vi "NN_Draw_Rectangle.vi"(4 "Clear":bool, 5 "font_size":sgl=20.0, 6 "Labels":string[](array[string])=["aeroplane", "bicycle", "bird", "boat", "bottle", "bus", "car", "cat", "chair", "cow", "diningtable", "dog", "horse", "motorbike", "person", "pottedplant", "sheep", "sofa", "train", "tvmonitor"], 7 "Border_Width":u32=4, 8 "error in (no error)":errorcluster, 9 "Colors":u32[](array[colorbox])=[6618880, 15679744, 16774656, 1740031, 13311, 33023, 52479, 65509, 65433, 65356, 65280, 5111552, 10092288, 15138560, 16763904, 16744192, 16724736, 16711680, 16711680, 16711680], 10 "Draw_Boxes":T1[](array[typedef]) {"BBox"."x" format="%#_4p"; "BBox"."y" format="%#_4p"; "BBox"."w" format="%#_4p"; "BBox"."h" format="%#_4p"}, 11 "Image_in":T3) -> (0 "error out":errorcluster, 1 "Exec_Time(s)":dbl=0.000148600014654221, 3 "Image_out":T3)   [LabVIEW 2020]
doc: "Draws bounding box regtangles around objects on the image based on BBox input information ."
uses:
  <vilib>/vision/Image Controls.llb/IMAQ Image.ctl
  <vilib>/Ngene/Deep Learning Toolkit/Toolkit/NN_Data/API/Data/Detection_Types/NN_BBox_Detection.ctl
  <vilib>/Ngene/Deep Learning Toolkit/Toolkit/NN_Data/API/Data/Detection_Types/NN_BBox.ctl
  <vilib>/Ngene/Deep Learning Toolkit/Toolkit/NN_Data/API/NN_Dims(C,H,W).ctl
  <vilib>/Ngene/Deep Learning Toolkit/Toolkit/Deep_Learning_Toolkit_by_Ngene.lvlib
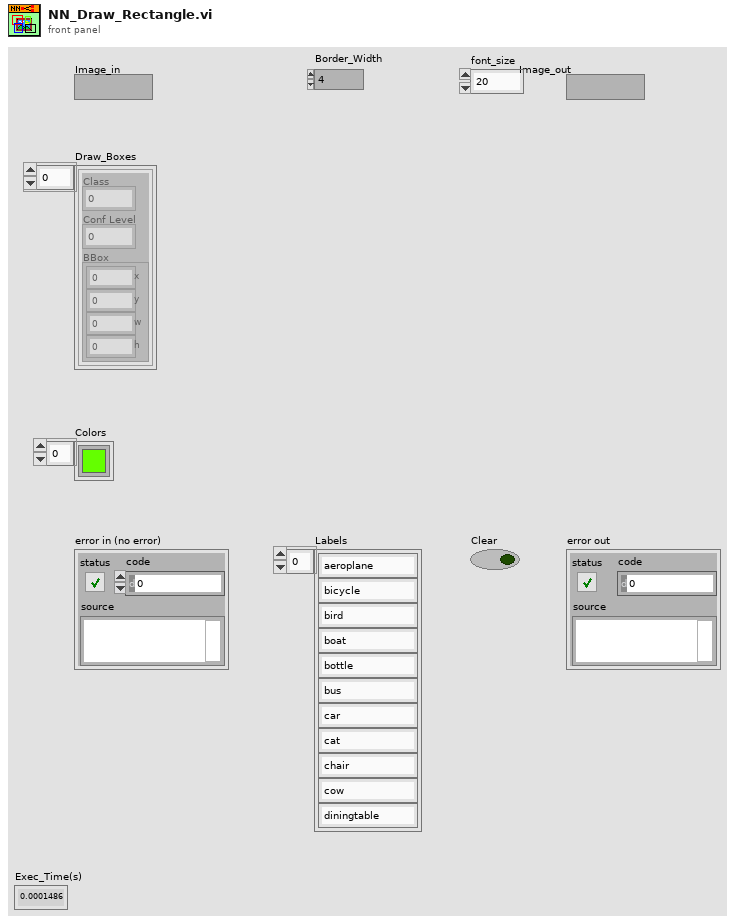
[diagram p1: front panel]
types:
  T1 = typedef "Deep_Learning_Toolkit_by_Ngene.lvlib/NN_BBox_Detection.ctl" = cluster{"Class":i32, "Conf Level":sgl, "BBox":T2}
  T2 = typedef "Deep_Learning_Toolkit_by_Ngene.lvlib/NN_BBox.ctl" = cluster{"x":sgl, "y":sgl, "w":sgl, "h":sgl}
  T3 = typedef "IMAQ Image.ctl" = refnum<image>
  T4 = typedef "Deep_Learning_Toolkit_by_Ngene.lvlib/NN_Dims(C,H,W).ctl" = cluster{"C":i32, "H":i32, "W":i32}
  T5 = cluster{"Desired Font (Application)":enum16{"User-specified Font", "Application Font", "System Font", "Dialog Font"}, "[User-specified Font]":cluster{"Font Name":string, "Size":i16, "Strikeout?":bool, "Italic?":bool, "Underline?":bool, "Outline?":bool, "Shadow?":bool, "Bold?":bool, "Rotation Angle":dbl}, "Horizontal Alignment":i16, "Vertical Alignment":i16}
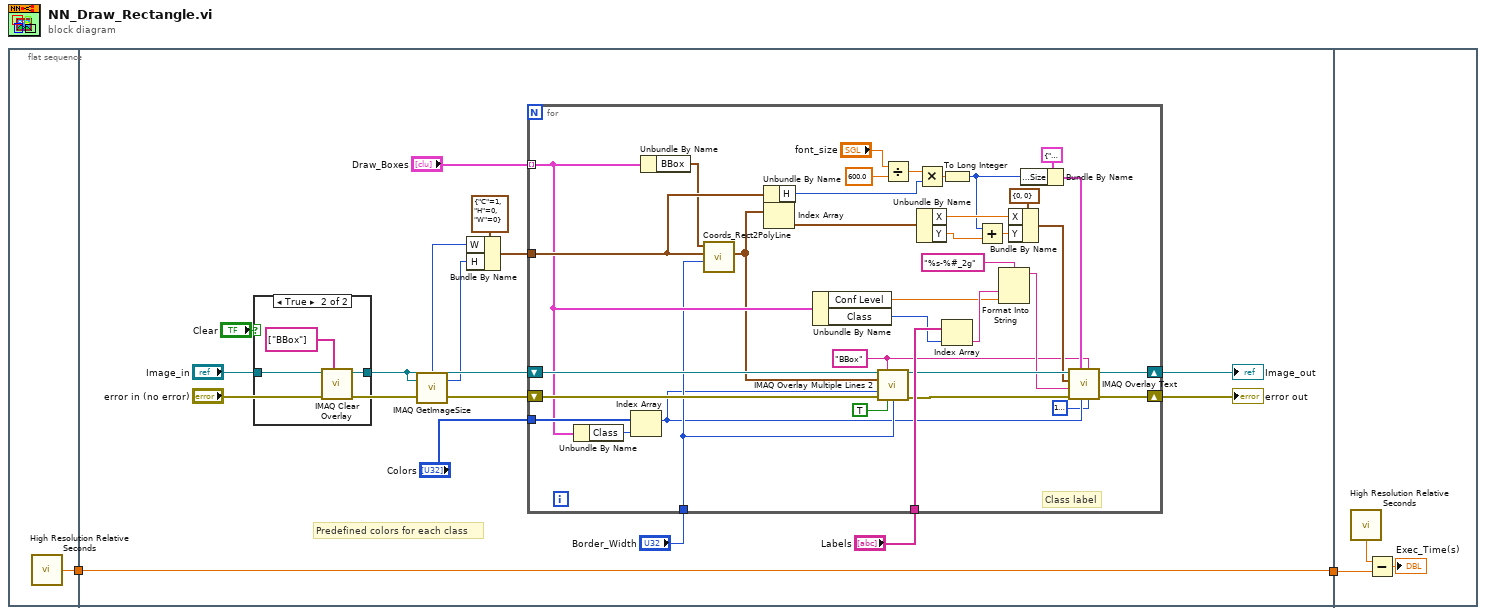
[diagram p0: block diagram]
diagram:
  n1 = flat-sequence {
    tunnel: [w3] -> w2
    tunnel: w2 -> [w9]
    tunnel: [w9] -> w1
    tunnel: w1 -> [w63]
    frame #0 {
      n2 = call <vilib>:"High Resolution Relative Seconds.vi"() -> ("relative seconds"=w3:dbl)
    }
    frame #1 {
      # "Predefined colors for each class"
      n3 = case shown="True" "Clear" {
        tunnel: "Image_in" -> [w20 w23]
        tunnel: [w20 w22] -> w12
        frame False {
        }
        frame True {
          n4 = call "IMAQ Clear Overlay"("Groups"=string[] ["BBox"], "Image"=w23) -> ("Image Out"=w22:T3)  [unwired: 8 in, 1 out]
        }
      }
      n5 = call "IMAQ GetImageSize"("Image"=w12, "error in (no error)"="error in (no error)") -> ("Y Resolution"=w10:i32, "X Resolution"=w11:i32, "error out"=w13:errorcluster)  [unwired: 2 in]
      n6 = Bundle By Name(cluster=T4 {"C"=1, "H"=0, "W"=0} ("In_Dims"), "W"=w11, "H"=w10) -> (w15:T4)
      n7 = for {
        tunnel: "Colors" -> [w60]
        shift-right: [w59] -> w19
        shift-left: w13 -> [w56]
        shift-right: [w58] -> w4
        shift-left: w12 -> [w55]
        tunnel: w15 -> [w57]
        tunnel: "Draw_Boxes" -> [w54] mode=indexing
        tunnel: "Border_Width" -> [w52]
        tunnel: "Labels" -> [w51]
        w36 = "BBox" ("Group")
        # "Class label"
        n8 = Unbundle By Name(w54) -> ("Class"=w53:i32)
        n9 = Index Array(array=w60, index=w53) -> (element=w25:u32)
        n10 = Unbundle By Name(w54) -> ("BBox"=w37:T2)
        n11 = call <vilib>:"Coords_Rect2PolyLine.vi"("Border_Width"=w52, "In_Dims"=w57, "BBox"=w37) -> ("PolyLine"=w30:cluster{"X":dbl, "Y":dbl}[])  [unwired: 8 in]
        n12 = Unbundle By Name(w57) -> ("H"=w31:i32)
        n13 = Index Array(array=w30) -> (element=w29:cluster{"X":dbl, "Y":dbl})  [unwired: 1 in]
        n14 = Unbundle By Name(w54) -> ("Conf Level"=w26:sgl, "Class"=w28:i32)
        n15 = call "IMAQ Overlay Multiple Lines 2"("Image"=w55, "Group"=w36, "Line End Points"=w30, "Color"=w25, "error in (no error)"=w56, "Maintain Width?"=TRUE, "Width"=w52) -> ("Image Out"=w50:T3, "error out"=w49:errorcluster)  [unwired: 7 in]
        n16 = Divide(x="font_size", y=sgl 600.0) -> (x/y=w39:sgl)
        n17 = Multiply(x=w39, y=w31) -> (x*y=w40:sgl)
        n18 = Unbundle By Name(w29) -> ("X"=w34:dbl, "Y"=w33:dbl)
        n19 = To Long Integer(number=w40) -> (32bit integer=w32:i32)
        n20 = Index Array(array=w51, index=w28) -> (element=w27:string)
        n21 = Add(x=w32, y=w33) -> (x+y=w46:dbl)
        n22 = Format Into String(format string="%s-%#_2g", w27, w26) -> (resulting string=w44:string)  [unwired: 2 in, 1 out]
        n23 = Bundle By Name(cluster=cluster{"X":i32, "Y":i32} {"X"=0, "Y"=0} ("Origin"), "X"=w34, "Y"=w46) -> (w47:cluster{"X":i32, "Y":i32})
        n24 = Bundle By Name(cluster=T5 {"Desired Font (Application)"=enum."User-specified Font", "[User-specified Font]"={"Font Name"="", "Size"=18, "Strikeout?"=FALSE, "Italic?"=FALSE, "Underline?"=FALSE, "Outline?"=FALSE, "Shadow?"=FALSE, "Bold?"=TRUE, "Rotation Angle"=0.0}, "Horizontal Alignment"=0, "Vertical Alignment"=0} ("Font, Size & Style"), "[User-specified Font].Size"=w32) -> (w42:T5)
        n25 = call "IMAQ Overlay Text"("BG Color (Transparent)"=u32 16777216, "Group"=w36, "Text Color (black)"=w25, "Font, Size & Style"=w42, "error in (no error)"=w49, "String"=w44, "Origin"=w47, "Image"=w50) -> ("error out"=w59:errorcluster, "Image Out"=w58:T3)  [unwired: 2 in]
      }
      "error out" <- w19
      "Image_out" <- w4
    }
    frame #2 {
      n26 = call <vilib>:"High Resolution Relative Seconds.vi"() -> ("relative seconds"=w62:dbl)
      n27 = Subtract(x=w62, y=w63) -> (x-y=→"Exec_Time(s)":dbl)
    }
  }
